vi "WS1050 Bench CAP Characterization.vi"() -> ()   [LabVIEW 2012]
panel:
  in  "Tab Control":enum32{"CONTROL", "INDICATION"}(tab)
  in  "RFFE Com Port":refnum<visa-resource-name>="COM3"
  in  "AD7747 Com Port":refnum<visa-resource-name>="COM1"
  in  "Init":bool=TRUE
  in  "Wafer":string="WS1050"
  in  "Lot":string="Toggle 7"
  in  "SN":string="01"
  in  "Temperature":string="RT"
  in  "Delay(ms)":u32=100
  in  "TMN DC\\CAP Data Log File Path":path=path "C:/Andy Tr/Temp"
  in  "String":string="WS1050 BENCH CAP CHARACTERIZATION"
  out "C3Cal (pF)":dbl=-4.9974111328125
  out "C1Cal (pF)":dbl=-4.5642919921875
  out "C2Cal (pF)":dbl=-4.9191376953125
  out "S_ValueC3(pF)":dbl=-4.9974111328125
  out "S_ValueC1(pF)":dbl=-4.5642919921875
  out "S_ValueC2(pF)":dbl=-4.9191376953125
  in  "Calib Socket":bool
  out "C1_Mesa(pF)":dbl
  out "C2_Mesa(pF)":dbl
  out "C3_Mesa(pF)":dbl
  in  "A364X_VDD":refnum<visa-resource-name>="GPIB1::6::INSTR"
  in  "IDD Limit":dbl=0.02 format="%.2p"
  in  "VDD":dbl=3.3
  in  "CP Setting":i32(ring) items=["CP OFF", "CP ON", "DVA OFF", "DVA ON", "ECAL OFF", "ECAL ON", "CP 40.25V", "CP 35V", "CP 38V", "CP 44V", "CP 50V", "CP 23.75V", "CP 25.25V", "CP 29.75V", "C1 ON", "C1 OFF", "C2 ON", "C2 OFF", "C3 ON", "C3 OFF"]
  in  "Send":bool
  in  "Init AD7747":bool
  out "C_min(pF)":string[](array[string])
  out "C_Max":string[](array[string])
  out "C_Min2(pF)":string[](array[string])
  out "error out":errorcluster
  in  "error in (no error)":errorcluster
  in  "stop":bool
  in  "Abort":bool
  in  "Start Test":bool
  out "Running loop":i32
  # "Company:  WiSpry Inc\n198 Fairbanks Ste 198 Irvine\n\nCreated by:  Andy V Tran\nDate:  03/11/2015\nTP:  WS1050 Bench\nCAP Characterization"
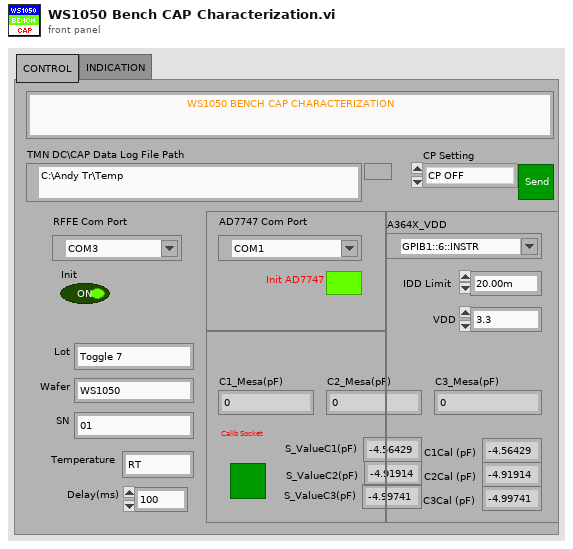
[diagram p1: front panel]
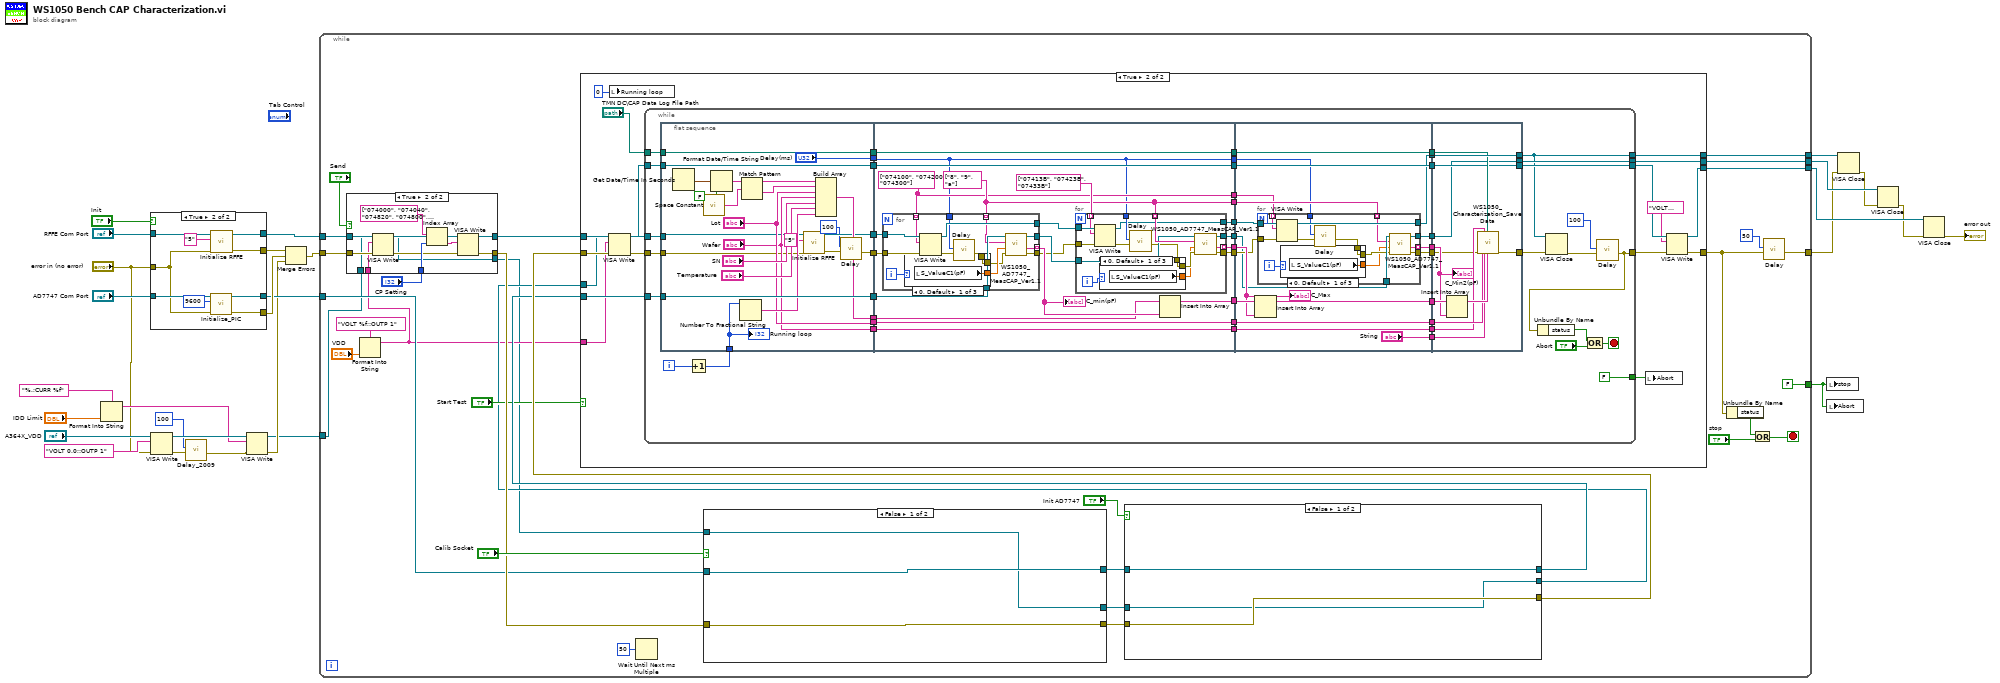
[diagram p0: block diagram]
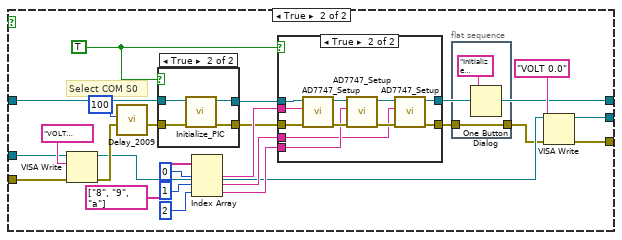
[diagram p3: hidden frame]
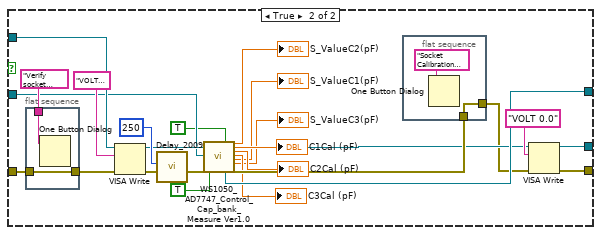
[diagram p6: hidden frame]
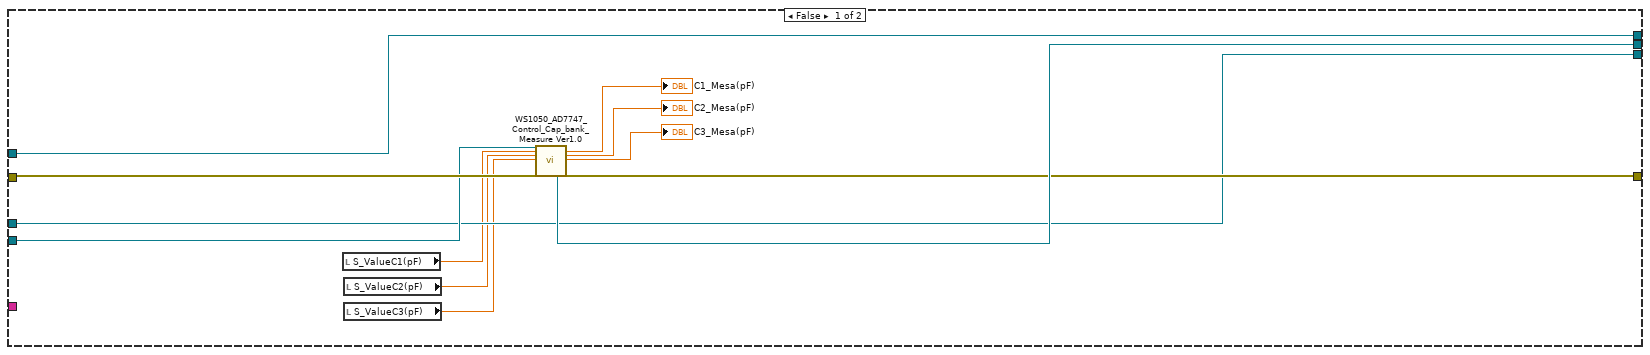
[diagram p7: hidden frame]
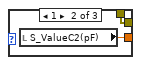
[diagram p8: hidden frame]
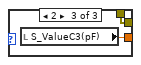
[diagram p9: hidden frame]
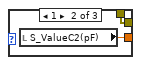
[diagram p10: hidden frame]
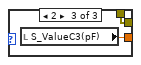
[diagram p11: hidden frame]
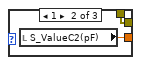
[diagram p12: hidden frame]
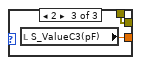
[diagram p13: hidden frame]
diagram:
  n1 = Format Into String(format string="%.;CURR %f", "IDD Limit") -> (resulting string=w18:string)  [unwired: 2 in, 1 out]
  n2 = case shown="True" "Init" {
    tunnel: "RFFE Com Port" -> [w31 w40]
    tunnel: [w31 w38] -> w27
    tunnel: "AD7747 Com Port" -> [w29 w36]
    tunnel: [w30 w35] -> w25
    tunnel: [w30 w34] -> w24
    tunnel: [w29 w33] -> w22
    tunnel: "error in (no error)" -> [w30 w32]
    frame False {
    }
    frame True {
      n3 = call "Initialize_PIC.vi"("error in (no error)"=w32, "baud rate"=u32 9600, "Select Com Port"=w36) -> ("error out"=w34:errorcluster, "VISA resource name out"=w33:refnum<visa-resource-name>)  [unwired: 7 in]
      n4 = call "Initialize RFFE.vi"("error in (no error)"=w32, "write buffer"="5", "Select Com Port"=w40) -> ("error out"=w35:errorcluster, "VISA resource name out"=w38:refnum<visa-resource-name>)  [unwired: 7 in]
    }
  }
  n5 = VISA Write(VISA resource name="A364X_VDD", write buffer="VOLT 0.0;:OUTP 1", error in (no error)="error in (no error)") -> (VISA resource name out=w19:refnum<visa-resource-name>, error out=w15:errorcluster)  [unwired: 1 out]
  n6 = call "Delay_2009.vi"("error in (no error)"=w15, "milliseconds to wait"=u32 100) -> ("error out"=w20:errorcluster)  [unwired: 9 in]
  n7 = VISA Write(VISA resource name=w19, write buffer=w18, error in (no error)=w20) -> (VISA resource name out=w9:refnum<visa-resource-name>, error out=w10:errorcluster)  [unwired: 1 out]
  n8 = Merge Errors(w25, w24, w10) -> (w23:errorcluster)
  n9 = while {
    tunnel: w27 -> [w69]
    tunnel: w23 -> [w70]
    tunnel: w22 -> [w57]
    tunnel: [w65] -> w5
    tunnel: [w63] -> w8
    tunnel: [w62] -> w7
    tunnel: w9 -> [w44]
    tunnel: [w48] -> w6
    tunnel: [FALSE ("stop")] -> w1
    stop <- w60 stop-if-true
    n10 = Format Into String(format string="VOLT %f;:OUTP 1", "VDD") -> (resulting string=w43:string)  [unwired: 2 in, 1 out]
    n11 = case shown="True" "Send" {
      tunnel: w70 -> [w370 w376]
      tunnel: [w370 w380] -> w58
      tunnel: [w369 w379] -> w68
      tunnel: "CP Setting" -> [_ w378]
      tunnel: w69 -> [w369 w377]
      tunnel: w44 -> [w368 w375]
      tunnel: w43 -> [_ w374]
      tunnel: [w368 w372] -> w42
      frame False {
      }
      frame True {
        n12 = VISA Write(VISA resource name=w375, write buffer=w374, error in (no error)=w376) -> (VISA resource name out=w372:refnum<visa-resource-name>, error out=w373:errorcluster)  [unwired: 1 out]
        n13 = Index Array(array=string[] ["074000", "074040", "074820", "074800", "074044", "074040", "074776", "07476F", "074773", "07477B", "07477C", "074760", "074762", "074768", "07413B", "074100", "07423B", "074200", "07433B", "074300"], index=w378) -> (element=w381:string)
        n14 = VISA Write(VISA resource name=w377, write buffer=w381, error in (no error)=w373) -> (VISA resource name out=w379:refnum<visa-resource-name>, error out=w380:errorcluster)  [unwired: 1 out]
      }
    }
    n15 = Wait Until Next ms Multiple(millisecond multiple=u32 50) -> ()  [unwired: 1 out]
    n16 = case shown="False" "Calib Socket" {
      tunnel: w58 -> [w123 w146]
      tunnel: [w123 w129] -> w52
      tunnel: w57 -> [w122 w127]
      tunnel: w42 -> [w121 w135]
      tunnel: [w121 w130] -> w53
      tunnel: [w122 w144] -> w51
      frame False {
      }
      frame True {
        n17 = flat-sequence {
          tunnel: [w149] -> w136
          tunnel: w146 -> [w149]
          tunnel: "Verify socket should be empty" ("message") -> [w148]
          frame #0 {
            n18 = One Button Dialog(message=w148) -> ()  [unwired: 1 in, 1 out]
          }
        }
        n19 = VISA Write(VISA resource name=w135, write buffer="VOLT 3.3;:OUTP 1", error in (no error)=w136) -> (VISA resource name out=w131:refnum<visa-resource-name>, error out=w133:errorcluster)  [unwired: 1 out]
        n20 = call "Delay_2009.vi"("error in (no error)"=w133, "milliseconds to wait"=u32 250) -> ("error out"=w126:errorcluster)  [unwired: 9 in]
        n21 = call "WS1050_AD7747_Control_Cap_bank_Measure Ver1.0.vi"("Select Com Port"=w127, "errorin"=w126, "Push Button to Measue Cap"=TRUE, "Push Button to Calibrate"=TRUE ("Push Button to Initialize AD7747")) -> ("Com Port Out"=w144:refnum<visa-resource-name>, "C2(pF)"=→"S_ValueC2(pF)":dbl, "C1_Mesa(pF)"=→"C1Cal (pF)":dbl, "C2_Mesa(pF)"=→"C2Cal (pF)":dbl, "C3_Mesa(pF)"=→"C3Cal (pF)":dbl, "C1(pF)"=→"S_ValueC1(pF)":dbl, "C3(pF)"=→"S_ValueC3(pF)":dbl, "error out"=w145:errorcluster)  [unwired: 16 in]
        n22 = flat-sequence {
          tunnel: [w150] -> w128
          tunnel: w145 -> [w150]
          frame #0 {
            n23 = One Button Dialog(message="Socket Calibration Completed, Please insert DUT into the Socket") -> ()  [unwired: 1 in, 1 out]
          }
        }
        n24 = VISA Write(VISA resource name=w131, write buffer="VOLT 0.0", error in (no error)=w128) -> (VISA resource name out=w130:refnum<visa-resource-name>, error out=w129:errorcluster)  [unwired: 1 out]
      }
    }
    n25 = case shown="False" "Init AD7747" {
      tunnel: w51 -> [w74 w99]
      tunnel: [w75 w79] -> w55
      tunnel: w52 -> [w75 w84]
      tunnel: [w74 w77] -> w54
      tunnel: w53 -> [w73 w85]
      tunnel: [w73 w80] -> w49
      frame False {
      }
      frame True {
        w89 = TRUE
        # "Select COM S0"
        n26 = VISA Write(VISA resource name=w85, write buffer="VOLT 3.3;:OUTP 1", error in (no error)=w84) -> (VISA resource name out=w81:refnum<visa-resource-name>, error out=w83:errorcluster)  [unwired: 1 out]
        n27 = call "Delay_2009.vi"("error in (no error)"=w83, "milliseconds to wait"=u32 100) -> ("error out"=w87:errorcluster)  [unwired: 9 in]
        n28 = case shown="True" w89 {
          tunnel: [w113 w118] -> w90
          tunnel: [w114 w117] -> w98
          tunnel: w99 -> [w114 w116]
          tunnel: w87 -> [w113 w115]
          frame False {
          }
          frame True {
            n29 = call "Initialize_PIC.vi"("error in (no error)"=w115, "Select Com Port"=w116) -> ("error out"=w118:errorcluster, "VISA resource name out"=w117:refnum<visa-resource-name>)  [unwired: 8 in]
          }
        }
        n30 = Index Array(array=string[] ["8", "9", "a"], index #1=0 ("index"), index #2=1 ("index"), index #3=2 ("index")) -> (element #1=w93:string, element #2=w92:string, element #3=w91:string)
        n31 = case shown="True" w89 {
          tunnel: w90 -> [w101 w104]
          tunnel: [w101 w102] -> w76
          tunnel: w98 -> [w100 w112]
          tunnel: w93 -> [_ w107]
          tunnel: w91 -> [_ w106]
          tunnel: w92 -> [_ w105]
          tunnel: [w100 w103] -> w77
          frame False {
          }
          frame True {
            n32 = call "AD7747_Setup.vi"("error in"=w104, "AD7747_Number"=w107, "Control"=w112) -> ("error out"=w111:errorcluster, "Control out"=w110:refnum<visa-resource-name>)  [unwired: 6 in, 1 out]
            n33 = call "AD7747_Setup.vi"("error in"=w111, "AD7747_Number"=w106, "Control"=w110) -> ("error out"=w109:errorcluster, "Control out"=w108:refnum<visa-resource-name>)  [unwired: 6 in, 1 out]
            n34 = call "AD7747_Setup.vi"("error in"=w109, "AD7747_Number"=w105, "Control"=w108) -> ("error out"=w102:errorcluster, "Control out"=w103:refnum<visa-resource-name>)  [unwired: 6 in, 1 out]
          }
        }
        n35 = flat-sequence {
          tunnel: w76 -> [w119]
          tunnel: [w119] -> w78
          frame #0 {
            n36 = One Button Dialog(message="Initialize AD7747 completed!") -> ()  [unwired: 1 in, 1 out]
          }
        }
        n37 = VISA Write(VISA resource name=w81, write buffer="VOLT 0.0", error in (no error)=w78) -> (VISA resource name out=w80:refnum<visa-resource-name>, error out=w79:errorcluster)  [unwired: 1 out]
      }
    }
    n38 = case shown="True" "Start Test" {
      tunnel: w68 -> [w156 w180]
      tunnel: w55 -> [w163 w175]
      tunnel: w54 -> [w162 w179]
      tunnel: [w160 w173] -> w66
      tunnel: [w156 w178] -> w63
      tunnel: [w161 w177] -> w62
      tunnel: w49 -> [w155 w174]
      tunnel: [w155 w170] -> w48
      tunnel: w43 -> [_ w165]
      frame False {
        n39 = local read "S_ValueC1(pF)"() -> (w154:dbl)
        n40 = local read "S_ValueC2(pF)"() -> (w153:dbl)
        n41 = local read "S_ValueC3(pF)"() -> (w152:dbl)
        n42 = call "WS1050_AD7747_Control_Cap_bank_Measure Ver1.0.vi"("Select Com Port"=w162, "S_Value C1"=w154, "S_Value C2"=w153, "S_Value C3"=w152, "errorin"=w163) -> ("Com Port Out"=w161:refnum<visa-resource-name>, "C1_Mesa(pF)"=→"C1_Mesa(pF)":dbl, "C2_Mesa(pF)"=→"C2_Mesa(pF)":dbl, "C3_Mesa(pF)"=→"C3_Mesa(pF)":dbl, "error out"=w160:errorcluster)  [unwired: 15 in, 3 out]
      }
      frame True {
        n43 = VISA Write(VISA resource name=w174, write buffer=w165, error in (no error)=w175) -> (VISA resource name out=w172:refnum<visa-resource-name>, error out=w176:errorcluster)  [unwired: 1 out]
        n44 = local write "Running loop"(0 ("Loop Running")) -> ()
        n45 = while {
          tunnel: w180 -> [w226]
          tunnel: w176 -> [w225]
          tunnel: w179 -> [w224]
          tunnel: [w181] -> w169
          tunnel: "TMN DC\\CAP Data Log File Path" -> [w218]
          tunnel: [w184] -> w178
          tunnel: [w214] -> w177
          tunnel: w172 -> [w210]
          tunnel: [w207] -> w171
          tunnel: [FALSE ("Abort")] -> w166
          i -> [w201]
          stop <- w221 stop-if-true
          n46 = flat-sequence {
            tunnel: w210 -> [w251]
            tunnel: w218 -> [w252]
            tunnel: w224 -> [w253]
            tunnel: w225 -> [w234]
            tunnel: w226 -> [w235]
            tunnel: [w231] -> w199
            tunnel: [w232] -> w198
            tunnel: [w253] -> w197
            tunnel: [w252] -> w196
            tunnel: [w251] -> w195
            tunnel: w194 -> [w238]
            tunnel: [w241] -> w193
            tunnel: ["Lot"] -> w192
            tunnel: ["Wafer"] -> w189
            tunnel: ["Delay(ms)"] -> w185
            tunnel: [w262] -> w229
            tunnel: [w268] -> w228
            tunnel: [w267] -> w223
            tunnel: [w266] -> w217
            tunnel: [w265] -> w215
            tunnel: [w264] -> w212
            tunnel: [w261] -> w208
            tunnel: [w260] -> w206
            tunnel: [w254] -> w205
            tunnel: [w259] -> w204
            tunnel: w199 -> [w274]
            tunnel: w198 -> [w273]
            tunnel: w197 -> [w270]
            tunnel: w196 -> [w264]
            tunnel: w195 -> [w261]
            tunnel: w193 -> [w257]
            tunnel: w192 -> [w256]
            tunnel: [w256] -> w191
            tunnel: w189 -> [w255]
            tunnel: [w255] -> w188
            tunnel: w185 -> [w254]
            tunnel: w229 -> [w334]
            tunnel: w228 -> [w333]
            tunnel: [w332] -> w227
            tunnel: w223 -> [w328]
            tunnel: [w329] -> w222
            tunnel: w217 -> [w324]
            tunnel: [w323] -> w216
            tunnel: w215 -> [w322]
            tunnel: [w331] -> w213
            tunnel: w212 -> [w331]
            tunnel: [w330] -> w209
            tunnel: w208 -> [w330]
            tunnel: w206 -> [w327]
            tunnel: w205 -> [w326]
            tunnel: w204 -> [w325]
            tunnel: [w321] -> w203
            tunnel: [w320] -> w202
            tunnel: w191 -> [w319]
            tunnel: [w319] -> w190
            tunnel: w188 -> [w318]
            tunnel: [w318] -> w187
            tunnel: ["String"] -> w186
            tunnel: w227 -> [w362]
            tunnel: w222 -> [w356]
            tunnel: [w367] -> w183
            tunnel: w216 -> [w366]
            tunnel: [w366] -> w184
            tunnel: [w363] -> w214
            tunnel: w213 -> [w365]
            tunnel: w209 -> [w364]
            tunnel: [w364] -> w207
            tunnel: w203 -> [w363]
            tunnel: w202 -> [w361]
            tunnel: w190 -> [w359]
            tunnel: w187 -> [w358]
            tunnel: w186 -> [w357]
            frame #0 {
              n47 = Get Date/Time In Seconds() -> (seconds since 1Jan1904=w247:timestamp)
              n48 = call <vilib>:"Space Constant.vi"() -> ("String"=w250:string)
              n49 = Format Date/Time String(seconds (now)=w247, UTC format=FALSE) -> (date/time string=w248:string)  [unwired: 1 out]
              n50 = Number To Fractional String(number=w238) -> (F-format string=w242:string)  [unwired: 3 in]
              n51 = Match Pattern(string=w248, regular expression=w250) -> (before substring=w246:string, after substring=w245:string)  [unwired: 3 out]
              n52 = call "Initialize RFFE.vi"("error in (no error)"=w234, "write buffer"="5", "Select Com Port"=w235) -> ("error out"=w233:errorcluster, "VISA resource name out"=w231:refnum<visa-resource-name>)  [unwired: 7 in]
              n53 = Build Array(w246, w245, "Lot", "Wafer", "SN", "Temperature", w242) -> (w241:string[])
              n54 = call "Delay.vi"("error in (no error)"=w233, "milliseconds to wait"=u32 100) -> ("error out"=w232:errorcluster)  [unwired: 9 in]
              "Running loop" <- w238
            }
            frame #1 {
              w260 = string[] ["8", "9", "a"]
              w259 = string[] ["074100", "074200", "074300"]
              n55 = for {
                tunnel: w274 -> [w310]
                tunnel: w273 -> [w309]
                tunnel: w259 -> [w308] mode=indexing
                tunnel: [w307] -> w271
                tunnel: w270 -> [w306]
                tunnel: [w305] -> w269
                tunnel: [w304] -> w258
                tunnel: w254 -> [w302]
                tunnel: w260 -> [w301] mode=indexing
                tunnel: [w300] -> w263 mode=indexing
                i -> [w299]
                n56 = VISA Write(VISA resource name=w310, write buffer=w308, error in (no error)=w309) -> (VISA resource name out=w307:refnum<visa-resource-name>, error out=w303:errorcluster)  [unwired: 1 out]
                n57 = call "Delay.vi"("error in (no error)"=w303, "milliseconds to wait"=w302) -> ("error out"=w297:errorcluster)  [unwired: 9 in]
                n58 = case shown="0, Default" w299 {
                  tunnel: [w312 w314 w316] -> w298
                  tunnel: w297 -> [w311 w313 w315]
                  tunnel: [w311 w313 w315] -> w296
                  frame 0, Default {
                    n59 = local read "S_ValueC1(pF)"() -> (w312:dbl)
                  }
                  frame 1 {
                    n60 = local read "S_ValueC2(pF)"() -> (w314:dbl)
                  }
                  frame 2 {
                    n61 = local read "S_ValueC3(pF)"() -> (w316:dbl)
                  }
                }
                n62 = call "WS1050_AD7747_MeasCAP_Ver1.1.vi"("error in (no error)"=w296, "OFFSet Cal"=w298, "AD7747_Number"=w301, "Control"=w306) -> ("error"=w304:errorcluster, "CAP (pF)"=w300:string, "Control out"=w305:refnum<visa-resource-name>)  [unwired: 4 in, 1 out]
              }
              "C_min(pF)" <- w263
              n63 = for {
                tunnel: w271 -> [w289]
                tunnel: w258 -> [w288]
                tunnel: string[] ["07413B", "07423B", "07433B"] -> [w287] mode=indexing
                tunnel: w254 -> [w285]
                tunnel: w260 -> [w284] mode=indexing
                tunnel: [w283] -> w267
                tunnel: [w282] -> w265
                tunnel: [w281] -> w266
                tunnel: w269 -> [w280]
                tunnel: [w279] -> w268 mode=indexing
                i -> [w277]
                n64 = VISA Write(VISA resource name=w289, write buffer=w287, error in (no error)=w288) -> (VISA resource name out=w281:refnum<visa-resource-name>, error out=w286:errorcluster)  [unwired: 1 out]
                n65 = call "Delay.vi"("error in (no error)"=w286, "milliseconds to wait"=w285) -> ("error out"=w276:errorcluster)  [unwired: 9 in]
                n66 = case shown="0, Default" w277 {
                  tunnel: [w291 w293 w295] -> w275
                  tunnel: w276 -> [w290 w292 w294]
                  tunnel: [w290 w292 w294] -> w278
                  frame 0, Default {
                    n67 = local read "S_ValueC1(pF)"() -> (w291:dbl)
                  }
                  frame 1 {
                    n68 = local read "S_ValueC2(pF)"() -> (w293:dbl)
                  }
                  frame 2 {
                    n69 = local read "S_ValueC3(pF)"() -> (w295:dbl)
                  }
                }
                n70 = call "WS1050_AD7747_MeasCAP_Ver1.1.vi"("error in (no error)"=w278, "OFFSet Cal"=w275, "AD7747_Number"=w284, "Control"=w280) -> ("error"=w283:errorcluster, "CAP (pF)"=w279:string, "Control out"=w282:refnum<visa-resource-name>)  [unwired: 4 in, 1 out]
              }
              n71 = Insert Into Array(array=w257, new element=w263) -> (w262:string[])  [unwired: 1 in]
            }
            frame #2 {
              n72 = Insert Into Array(array=w334, new element=w333) -> (w332:string[])  [unwired: 1 in]
              n73 = for {
                tunnel: w324 -> [w349]
                tunnel: w328 -> [w348]
                tunnel: w325 -> [w347] mode=indexing
                tunnel: [w346] -> w323
                tunnel: w322 -> [w345]
                tunnel: [w344] -> w321
                tunnel: [w343] -> w329
                tunnel: w326 -> [w341]
                tunnel: w327 -> [w340] mode=indexing
                tunnel: [w339] -> w320 mode=indexing
                i -> [w338]
                n74 = VISA Write(VISA resource name=w349, write buffer=w347, error in (no error)=w348) -> (VISA resource name out=w346:refnum<visa-resource-name>, error out=w342:errorcluster)  [unwired: 1 out]
                n75 = call "Delay.vi"("error in (no error)"=w342, "milliseconds to wait"=w341) -> ("error out"=w336:errorcluster)  [unwired: 9 in]
                n76 = case shown="0, Default" w338 {
                  tunnel: [w351 w353 w355] -> w335
                  tunnel: w336 -> [w350 w352 w354]
                  tunnel: [w350 w352 w354] -> w337
                  frame 0, Default {
                    n77 = local read "S_ValueC1(pF)"() -> (w351:dbl)
                  }
                  frame 1 {
                    n78 = local read "S_ValueC2(pF)"() -> (w353:dbl)
                  }
                  frame 2 {
                    n79 = local read "S_ValueC3(pF)"() -> (w355:dbl)
                  }
                }
                n80 = call "WS1050_AD7747_MeasCAP_Ver1.1.vi"("error in (no error)"=w337, "OFFSet Cal"=w335, "AD7747_Number"=w340, "Control"=w345) -> ("error"=w343:errorcluster, "CAP (pF)"=w339:string, "Control out"=w344:refnum<visa-resource-name>)  [unwired: 4 in, 1 out]
              }
              "C_Max" <- w333
            }
            frame #3 {
              n81 = Insert Into Array(array=w362, new element=w361) -> (w360:string[])  [unwired: 1 in]
              n82 = call "WS1050_Characterization_Save Data.vi"("error in (no error)"=w356, "Lot"=w359, "Wafer"=w358, "TP"=w357, "TMN DC\\CAP Data Log File Path"=w365, "All Out"=w360) -> ("error out"=w367:errorcluster)  [unwired: 19 in, 2 out]
              "C_Min2(pF)" <- w361
            }
          }
          n83 = Increment(x=w201) -> (x+1=w194:i32)
          n84 = VISA Close(VISA resource name=w184, error in (no error)=w183) -> (error out=w182:errorcluster)
          n85 = call "Delay.vi"("error in (no error)"=w182, "milliseconds to wait"=u32 100) -> ("error out"=w181:errorcluster)  [unwired: 9 in]
          n86 = Unbundle By Name(w181) -> ("status"=w220:bool)
          n87 = Or(x=w220, y="Abort") -> (x .or. y?=w221:bool)
        }
        n88 = local write "Abort"(w166) -> ()
        n89 = VISA Write(VISA resource name=w171, write buffer="VOLT 0.0;:OUTP 0", error in (no error)=w169) -> (VISA resource name out=w170:refnum<visa-resource-name>, error out=w173:errorcluster)  [unwired: 1 out]
      }
    }
    n90 = Unbundle By Name(w66) -> ("status"=w67:bool)
    n91 = Or(x=w67, y="stop") -> (x .or. y?=w60:bool)
    n92 = call "Delay.vi"("error in (no error)"=w66, "milliseconds to wait"=u32 50) -> ("error out"=w65:errorcluster)  [unwired: 9 in]
  }
  n93 = local write "stop"(w1) -> ()
  n94 = local write "Abort"(w1) -> ()
  n95 = VISA Close(VISA resource name=w8, error in (no error)=w5) -> (error out=w4:errorcluster)
  n96 = VISA Close(VISA resource name=w7, error in (no error)=w4) -> (error out=w3:errorcluster)
  n97 = VISA Close(VISA resource name=w6, error in (no error)=w3) -> (error out=→"error out":errorcluster)
